vi "subParseForLayersAndComponents.vi"(8 "error in (no error)":errorcluster, 9 "Parent node":string, 11 "Refnum in":refnum<k20>) -> (0 "error out":errorcluster, 1 "Rules":T1, 3 "Refnum out":refnum<k20>)   [LabVIEW 2020, in "DefaultExtensions.lvlib" / "CDefaultRuleFileParser.lvclass"]
uses:
  CDefaultRuleFileParser.lvclass
  obj/Addons/ExtensionInterfaces.lvlibp/IRuleFileParser/RulesDefinition.ctl
  obj/Addons/ExtensionInterfaces.lvlibp/IRuleFileParser/IRuleFileParser.lvclass
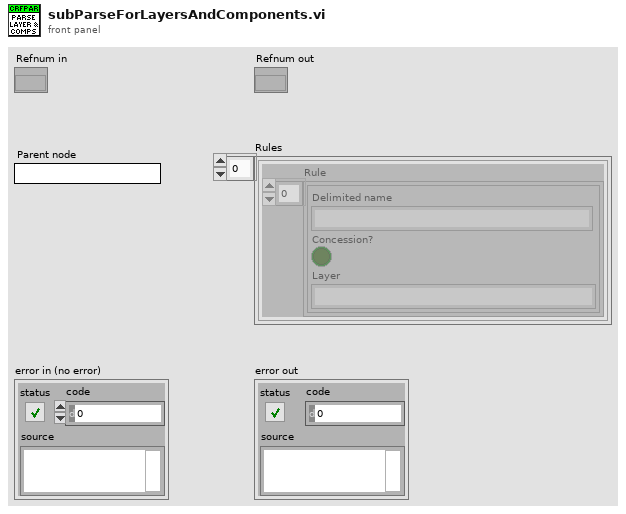
[diagram p1: front panel]
types:
  T1 = typedef "ExtensionInterfaces.lvlibp/IRuleFileParser.lvclass/RulesDefinition.ctl" = cluster{"Rule":cluster{"Delimited name":string, "Concession?":bool, "Layer":string}[]}[]
  T2 = cluster{cluster{"Delimited name":string, "Concession?":bool, "Layer":string}[]}[]
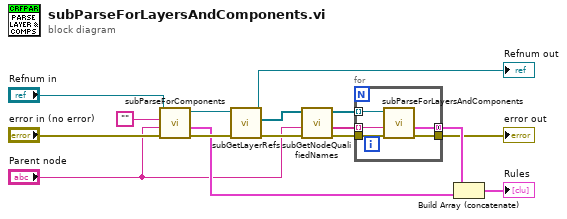
[diagram p0: block diagram]
diagram:
  n1 = call "subParseForComponents.vi"("error in (no error)"="error in (no error)", "Parent layer"="Parent node", "Parent component"="", "Refnum in"="Refnum in") -> ("error out"=w11:errorcluster, "Rules"=w6:T2, "Refnum out"=w12:refnum<k20>)  [unwired: 5 in]
  n2 = call "subGetLayerRefs.vi"("error in (no error)"=w11, "Refnum in"=w12) -> ("error out"=w15:errorcluster, "node result array"=w16:refnum<k20>[], "Refnum out"=→"Refnum out":refnum<k20>)  [unwired: 7 in]
  n3 = call "subGetNodeQualifiedNames.vi"("error in (no error)"=w15, "Parent node"="Parent node", "node[] in"=w16) -> ("error out"=w8:errorcluster, "node name[]"=w9:string[], "node[]"=w10:refnum<k20>[])  [unwired: 6 in]
  n4 = for {
    tunnel: w10 -> [w21] mode=indexing
    tunnel: w9 -> [w20] mode=indexing
    tunnel: w8 -> [w19]
    tunnel: [w18] -> w7 mode=concatenating
    tunnel: [w17] -> w4
    n5 = call "subParseForLayersAndComponents.vi"("error in (no error)"=w19, "Parent node"=w20, "Refnum in"=w21) -> ("error out"=w17:errorcluster, "Rules"=w18:T1)  [unwired: 6 in, 1 out]
  }
  "error out" <- w4
  n6 = Build Array (concatenate)(w7, w6) -> (→"Rules":T1)
